vi "Insert Node.vi"(5 "Path to LabVIEW File":path, 6 "Variant in":variant, 7 "Shift Pressed?":bool, 8 "error in (no error)":errorcluster, 10 "QD Combo Box Ref":refnum<vi>, 11 "Selection List[]":refnum<vi>[](array[refnum])) -> (0 "error out":errorcluster, 3 "element":refnum<vi>, 4 "Variant out":variant)   [LabVIEW 2021, in "Migrator Reusables.lvlib"]
doc: "Inserts the object specified by name in the Quick Drop dialog box on the selected wire(s) on the diagram. If [Shift] is also pressed, and multiple wires were selected, a single instance of the object is inserted on those wires.\n\nDefault Shortcut - [I]"
uses:
  Migrator Reusables.lvlib
  <vilib>/Utility/miscctls.llb/LVPositionTypeDef.ctl
  <vilib>/Utility/miscctls.llb/LVPointTypeDef.ctl
  55ef8f48-70f1-403b-b4c9-42cfcc39d2a5.vi
  a401b57f-dff2-4459-b358-16b2136f329f.vi
  <vilib>/Comparison/Less/Less Functor/Less Functor.lvclass
panel:
  in  "Palette Object Name":string
  in  "Select a VI":string="Select a VI..."
  in  "Undo Name":string="Insert"
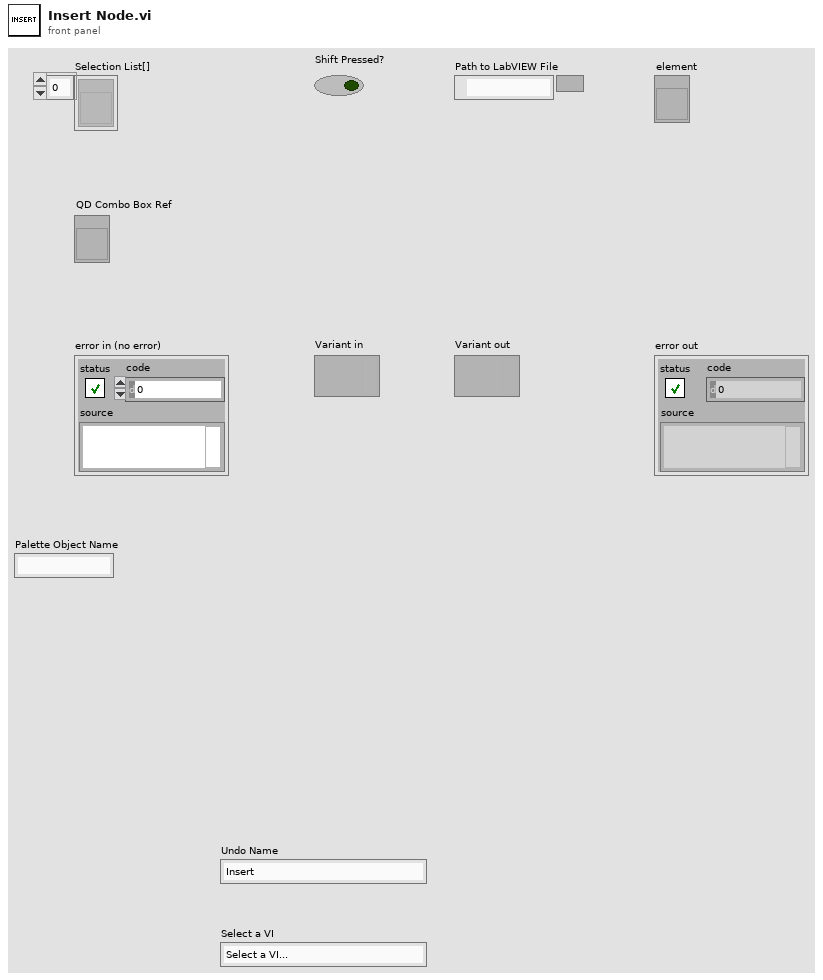
[diagram p1: front panel]
types:
  T1 = cluster{"Not Error Wire?":bool, "Source Term Top":i32, "Source Term Left":i32, "Wire Ref":refnum<vi>, "Source Term":refnum<vi>, "Sink Terms":refnum<vi>[], "Tried this one yet?":bool, "Sink Term Owner Owners":refnum<vi>[]}
  T2 = typedef "LVPositionTypeDef.ctl" = cluster{"Left":i32, "Top":i32}
  T3 = typedef "LVPointTypeDef.ctl" = cluster{"Horizontal":i16, "Vertical":i16}
  T4 = cluster{"Not Error Wire?":bool, "Source Term Top":i32, "Source Term Left":i32, "Wire Ref":refnum<vi>, "Source Term":refnum<vi>, "Sink Terms":refnum<vi>[], "Tried this one yet?":bool, "Sink Term Owner Owners":refnum<vi>[]}[]
  T5 = cluster{"Position":cluster{"h":i16, "v":i16}, "Flags":i32, "Type":enum32{"LooseEnd", "Endpoint", "Bend", "Junction"}, "Up Joint Index":i16, "Down Joint Index":i16, "Left Joint Index":i16, "Right Joint Index":i16}[]
  T6 = cluster{"Position":cluster{"h":i16, "v":i16}, "Flags":i32, "Type":enum32{"LooseEnd", "Endpoint", "Bend", "Junction"}, "Up Joint Index":i16, "Down Joint Index":i16, "Left Joint Index":i16, "Right Joint Index":i16}
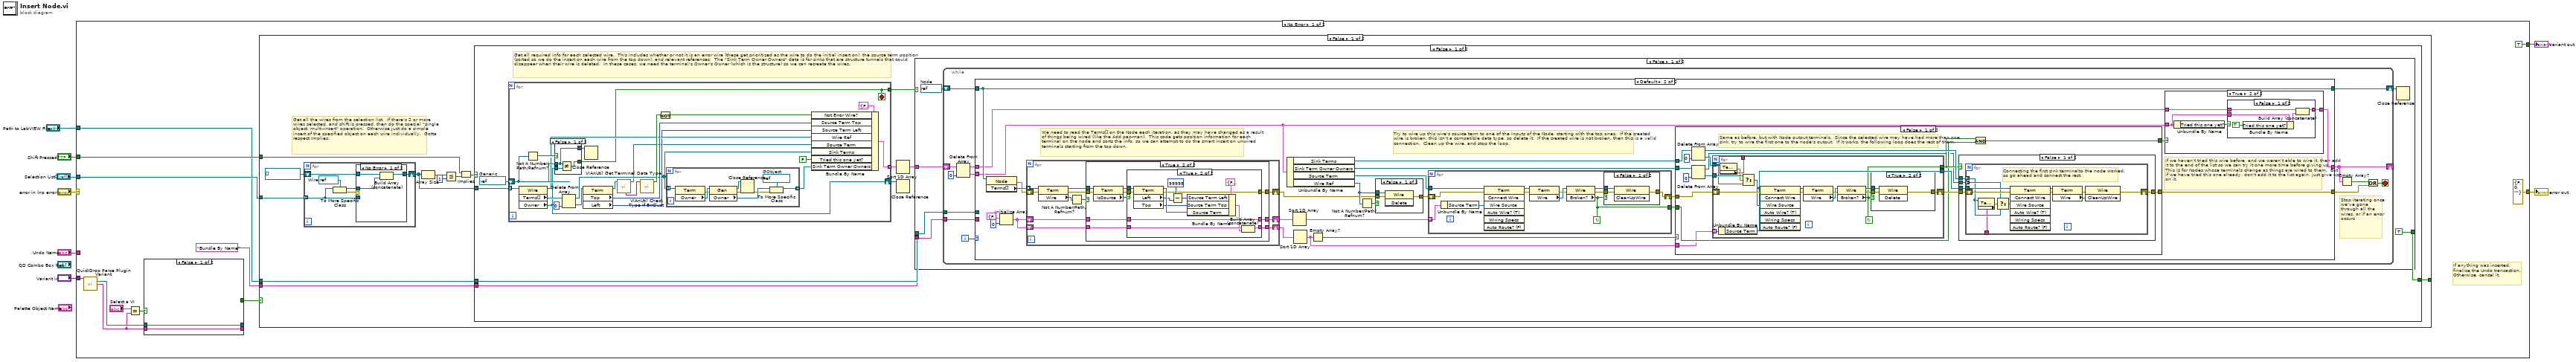
[diagram p0: block diagram]
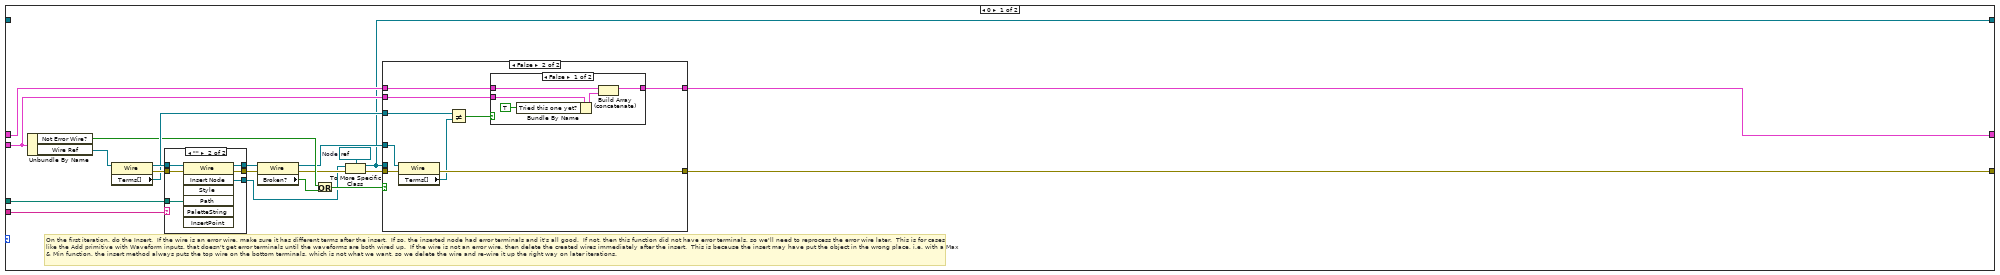
[diagram p2: hidden frame]
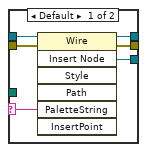
[diagram p3: hidden frame]
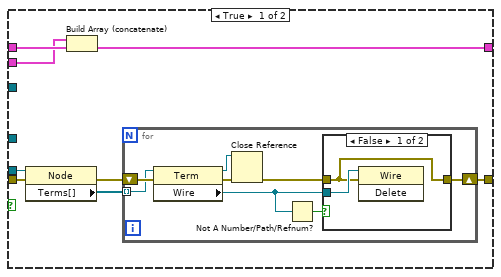
[diagram p4: hidden frame]
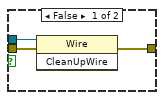
[diagram p9: hidden frame]
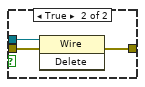
[diagram p13: hidden frame]
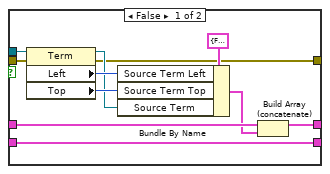
[diagram p15: hidden frame]
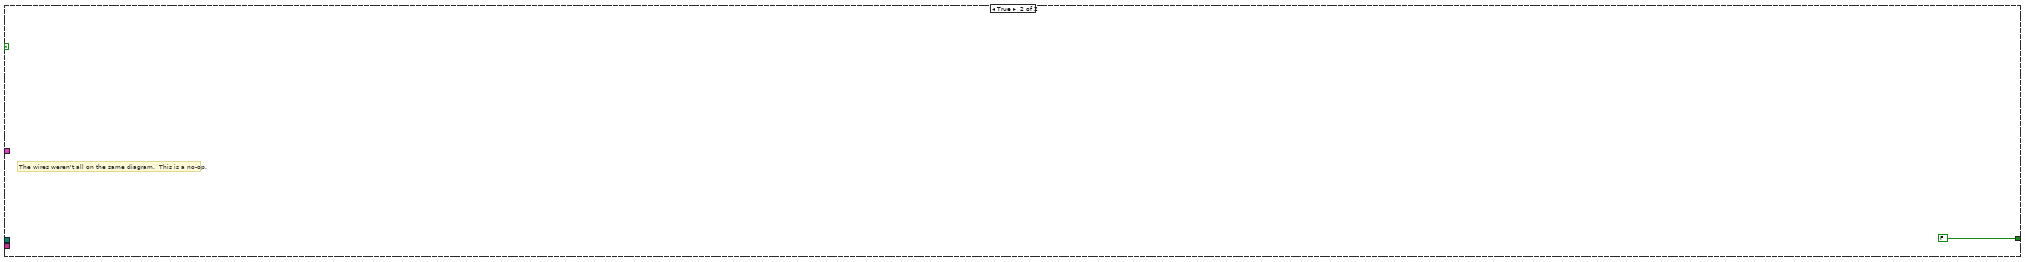
[diagram p16: hidden frame]
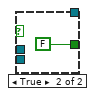
[diagram p17: hidden frame]
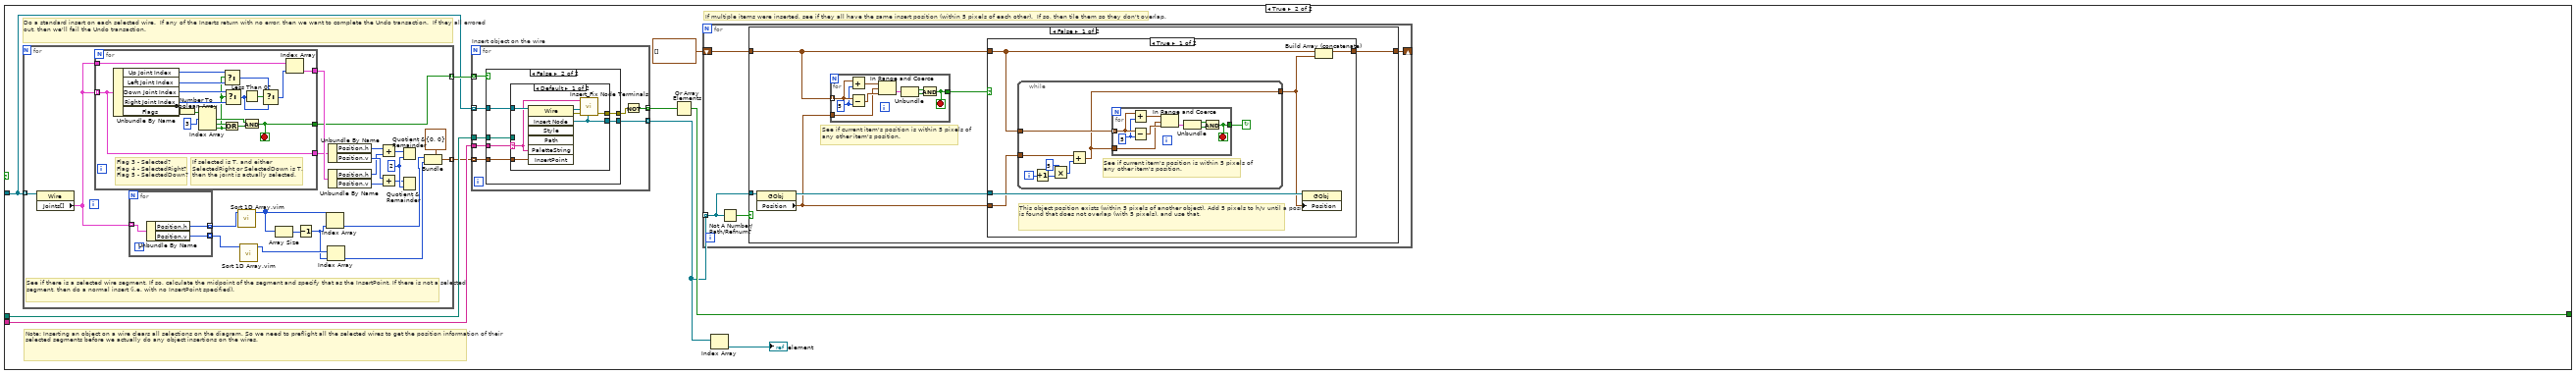
[diagram p18: hidden frame]
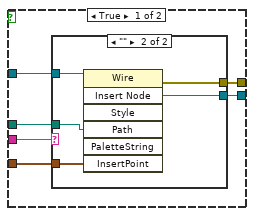
[diagram p19: hidden frame]
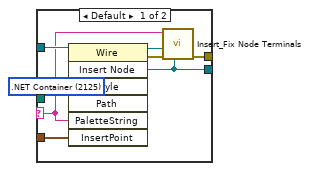
[diagram p20: hidden frame]
diagram:
  n1 = case shown="No Error" "error in (no error)" {
    selector: "error in (no error)" -> [_ w486]
    tunnel: [errorcluster {"status"=FALSE, "code"=0, "source"=""} ("error IO") w486] -> w7
    tunnel: "Shift Pressed?" -> [w18 _]
    tunnel: "Variant in" -> [w20 _]
    tunnel: "Undo Name" -> [_ _]
    tunnel: [TRUE _] -> w3
    tunnel: "Selection List[]" -> [w12 _]
    tunnel: "Path to LabVIEW File" -> [w9 _]
    frame No Error {
      # "If anything was inserted, finalize the Undo transaction.  Otherwise, cancel it."
      n2 = call <vilib>:"QuickDrop Parse Plugin Variant.vi"("QDKS Variant in"=w20) -> ("Project VI Path"=w15:path, "Palette Object Name"=w14:string)  [unwired: 12 in, 1 out]
      n3 = Equal?(x="Select a VI", y=w14) -> (x = y?=w16:bool)
      n4 = case shown="False" w16 {
        tunnel: w14 -> [w483 _]
        tunnel: w15 -> [w482 _]
        tunnel: [w483 _] -> _
        tunnel: [w482 w484] -> _
        tunnel: [_ w485] -> w13
        frame False {
        }
        frame True {
          # "NEW IN 2015: Catching \"Select a VI...\" and offering a file dialog to pick a VI to insert from disk."
          n5 = call <vilib>:"File Dialog - LabVIEW Files.vi"() -> ("cancelled"=w485:bool, "Path to LabVIEW File"=w484:path)  [unwired: 10 in]
        }
      }
      n6 = case shown="False" w13 {
        tunnel: w12 -> [w31 _]
        tunnel: w18 -> [w26 _]
        tunnel: [w23 _] -> _
        tunnel: w9 -> [w22 _]
        tunnel: "Bundle By Name" ("Palette Object Name") -> [w21 _]
        frame False {
          # "Get all the wires from the selection list.  If there's 2 or more wires selected, and shift is pressed, then do the special \"single object, multi-insert\" operation.  Otherwise just do a simple insert of the specified object on each wire individually.  Gotta respect Implies."
          n7 = for {
            tunnel: w31 -> [w473] mode=indexing
            shift-right: [w472] -> w25
            shift-left: refnum<vi>[] [] -> [w474]
            w476 = refnum<vi> refnum  # Wire
            n8 = To More Specific Class(target class=w476, reference=w473) -> (specific class reference=w471:refnum<vi>, error out=w475:errorcluster)  [unwired: 1 in]
            n9 = case shown="No Error" w475 {
              tunnel: w474 -> [w479 w481]
              tunnel: w473 -> [_ w480]
              tunnel: [w478 w481] -> w472
              tunnel: w471 -> [w477 _]
              frame No Error {
                n10 = Build Array (concatenate)(w479, w477) -> (w478:refnum<vi>[])
              }
              frame Error {
                n11 = Close Reference(reference=w480) -> ()  [unwired: 1 in, 1 out]
              }
            }
          }
          n12 = Array Size(array=w25) -> (size(s)=w29:i32)
          n13 = Less Or Equal?(x=w29, y=1) -> (x <= y?=w27:bool)
          n14 = Implies(1:w27, 2:w26) -> (0:w24:bool)
          n15 = case shown="False" w24 {
            tunnel: w21 -> [w33 w334]
            tunnel: w22 -> [w34 w333]
            tunnel: w25 -> [w36 w332]
            tunnel: [w32 w330] -> w23
            frame False {
              w39 = refnum<vi> refnum  # Generic
              # "Get all required info for each selected wire.  This includes whether or not it is an error wire (these get prioritized as the wire to do the initial insert on), the source term position (sorted so we do the insert on each wire from the top down), and relevant references.  The \"Sink Term Owner Owners\" data is for sinks that are structure tunnels that could disappear when their wire is deleted.  In these cases, we need the terminal's Owner's Owner (which is the structure) so we can recreate the wires."
              n16 = for {
                shift-right: [w298] -> w40
                shift-left: w39 -> [w313]
                tunnel: [w299] -> w38
                tunnel: w36 -> [w302] mode=indexing
                tunnel: [w301] -> w35 mode=indexing
                stop <- w299 stop-if-true
                n17 = property class="Wire"(reference=w302) -> (reference out=w305:refnum<vi>, "Terms[]"=w312:refnum<vi>[], "Owner"=w298:refnum<vi>)  [unwired: 1 in, 1 out]
                n18 = Not A Number/Path/Refnum?(number/path/refnum=w313) -> (NaN/Path/Refnum?=w310:bool)
                n19 = case shown="False" w310 {
                  tunnel: [w324 FALSE] -> w299
                  tunnel: w298 -> [w325 _]
                  tunnel: w313 -> [w323 _]
                  tunnel: [w323 _] -> w295
                  frame False {
                    n20 = Not Equal?(x=w323, y=w325) -> (x != y?=w324:bool)
                  }
                  frame True {
                  }
                }
                n21 = Delete From Array(array=w312, index=0) -> (deleted portion=w300:refnum<vi>, array with subset deleted=w297:refnum<vi>[])  [unwired: 1 in]
                n22 = property class="Term"(reference=w300) -> (reference out=w294:refnum<vi>, "Top"=w307:i32, "Left"=w296:i32)  [unwired: 1 in, 1 out]
                n23 = Close Reference(reference=w295) -> ()  [unwired: 1 in, 1 out]
                n24 = call <vilib>:"VIAnUtil Get Terminal Data Type.vi"("Terminal in"=w294) -> ("Terminal out"=w293:refnum<vi>, "Type Variant"=w292:variant)  [unwired: 7 in, 2 out]
                n25 = call <vilib>:"VIAnUtil Check Type If ErrClust.vi"("Data In"=w292) -> ("IsErrClust?"=w308:bool)  [unwired: 1 in, 9 out]
                n26 = Not(x=w308) -> (.not. x?=w306:bool)
                n27 = for {
                  tunnel: w297 -> [w322] mode=indexing
                  tunnel: [w319] -> w303 mode=indexing
                  w318 = refnum<vi> refnum  # GObject
                  n28 = property class="Term"(reference=w322) -> (error out=w317:errorcluster, "Owner"=w321:refnum<vi>)  [unwired: 1 in, 1 out]
                  n29 = property class="Gen"(reference=w321, error in=w317) -> (reference out=w315:refnum<vi>, error out=w316:errorcluster, "Owner"=w320:refnum<vi>)
                  n30 = Close Reference(reference=w315, error in (no error)=w316) -> (error out=w314:errorcluster)
                  n31 = To More Specific Class(target class=w318, reference=w320, error in=w314) -> (specific class reference=w319:refnum<vi>)  [unwired: 1 out]
                }
                n32 = Bundle By Name(cluster=T1 {"Not Error Wire?"=FALSE, "Source Term Top"=0, "Source Term Left"=0, "Wire Ref"=refnum, "Source Term"=refnum, "Sink Terms"=[], "Tried this one yet?"=FALSE, "Sink Term Owner Owners"=[]} ("Wire Information"), "Not Error Wire?"=w306, "Source Term Top"=w307, "Source Term Left"=w296, "Wire Ref"=w305, "Source Term"=w293, "Sink Terms"=w297, "Tried this one yet?"=FALSE, "Sink Term Owner Owners"=w303) -> (w301:T1)
              }
              n33 = Sort 1D Array(array=w35) -> (sorted array=w37:T4)
              n34 = Close Reference(reference=w40) -> ()  [unwired: 1 in, 1 out]
              n35 = case shown="False" w38 {
                tunnel: w37 -> [w46 _]
                tunnel: w33 -> [w43 _]
                tunnel: w34 -> [w42 _]
                tunnel: [TRUE FALSE] -> w32
                frame False {
                  w45 = refnum<vi> refnum  # Node
                  n36 = while {
                    shift-right: [w57] -> _
                    shift-left: w46 -> [w54]
                    shift-right: [w48] -> w44
                    shift-left: w45 -> [w56]
                    tunnel: w43 -> [w50]
                    tunnel: w42 -> [w49]
                    i -> [w58]
                    stop <- w51 stop-if-true
                    # "Stop iterating once we've gone through all the wires, or if an error occurs"
                    n37 = Delete From Array(array=w54, index=0) -> (deleted portion=w59:T1, array with subset deleted=w53:T4)  [unwired: 1 in]
                    n38 = case shown="Default" w58 {
                      tunnel: w59 -> [w79 w136]
                      tunnel: w53 -> [w67 w143]
                      tunnel: [w60 w151] -> w48
                      tunnel: [w80 w142] -> w57
                      tunnel: w56 -> [_ w151]
                      tunnel: [w78 w146] -> w47
                      tunnel: w50 -> [w65 _]
                      tunnel: w49 -> [w66 _]
                      frame 0 {
                        w63 = refnum<vi> refnum  # Node
                        # "On the first iteration, do the Insert.  If the wire is an error wire, make sure it has different terms after the insert.  If so, the inserted node had error terminals and it's all good.  If not, then this function did not have error terminals, so we'll need to reprocess the error wire later.  This is for cases like the Add primitive with Waveform inputs, that doesn't get error terminals until the waveforms are both wired up.  If the wire is not an error wire, then delete the created wires immediately after the insert.  This is because the insert may have put the object in the wrong place, i.e. with a Max & Min function, the insert method always puts the top wire on the bottom terminals, which is not what we want, so we delete the wire and re-wire it up the right way on later iterations."
                        n39 = Unbundle By Name(w79) -> ("Not Error Wire?"=w73:bool, "Wire Ref"=w77:refnum<vi>)
                        n40 = property class="Wire"(reference=w77) -> (reference out=w75:refnum<vi>, error out=w76:errorcluster, "Terms[]"=w74:refnum<vi>[])  [unwired: 1 in]
                        n41 = case shown="\"\"" w65 {
                          selector: w65 -> [w81 _]
                          tunnel: [w86 w92] -> w61
                          tunnel: w76 -> [w85 w91]
                          tunnel: w75 -> [w84 w90]
                          tunnel: [w83 w89] -> w72
                          tunnel: [w82 w88] -> w71
                          tunnel: w66 -> [_ w87]
                          frame Default {
                            n42 = invoke class="Wire" method="Insert Node"(reference=w84, error in=w85, "PaletteString"=w81) -> (reference out=w83:refnum<vi>, error out=w82:errorcluster, "Insert Node"=w86:refnum<vi>)  [unwired: 4 in, 4 out]
                          }
                          frame "" {
                            n43 = invoke class="Wire" method="Insert Node"(reference=w90, error in=w91, "Path"=w87) -> (reference out=w89:refnum<vi>, error out=w88:errorcluster, "Insert Node"=w92:refnum<vi>)  [unwired: 4 in, 4 out]
                          }
                        }
                        n44 = property class="Wire"(reference=w72, error in=w71) -> (reference out=w70:refnum<vi>, error out=w64:errorcluster, "Broken?"=w69:bool)
                        n45 = Or(x=w73, y=w69) -> (x .or. y?=w68:bool)
                        n46 = To More Specific Class(target class=w63, reference=w61, error in=w64) -> (specific class reference=w60:refnum<vi>, error out=w62:errorcluster)
                        n47 = case shown="False" w68 {
                          tunnel: w67 -> [w100 w120]
                          tunnel: [w98 w119] -> w80
                          tunnel: w79 -> [w99 w118]
                          tunnel: [w93 w115] -> w78
                          tunnel: w62 -> [w95 w117]
                          tunnel: w70 -> [_ w116]
                          tunnel: w74 -> [_ w113]
                          tunnel: w60 -> [w96 _]
                          frame True {
                            n48 = property class="Node"(reference=w96, error in=w95) -> (error out=w97:errorcluster, "Terms[]"=w94:refnum<vi>[])  [unwired: 1 out]
                            n49 = Build Array (concatenate)(w99, w100) -> (w98:T4)
                            n50 = for {
                              shift-right: [w102] -> w93
                              shift-left: w97 -> [w108]
                              tunnel: w94 -> [w107] mode=indexing
                              n51 = property class="Term"(reference=w107, error in=w108) -> (reference out=w105:refnum<vi>, error out=w106:errorcluster, "Wire"=w101:refnum<vi>)
                              n52 = Close Reference(reference=w105, error in (no error)=w106) -> (error out=w103:errorcluster)
                              n53 = Not A Number/Path/Refnum?(number/path/refnum=w101) -> (NaN/Path/Refnum?=w104:bool)
                              n54 = case shown="False" w104 {
                                tunnel: w103 -> [w109 w111]
                                tunnel: [w109 w111] -> w102
                                tunnel: w101 -> [w110 _]
                                frame False {
                                n55 = invoke class="Wire" method="Delete"(reference=w110, error in=w109) -> ()  [unwired: 1 in, 3 out]
                                }
                                frame True {
                                }
                              }
                            }
                          }
                          frame False {
                            n56 = property class="Wire"(reference=w116, error in=w117) -> (error out=w115:errorcluster, "Terms[]"=w114:refnum<vi>[])  [unwired: 1 out]
                            n57 = Not Equal?(x=w113, y=w114) -> (x != y?=w112:bool)
                            n58 = case shown="False" w112 {
                              tunnel: w120 -> [w125 w126]
                              tunnel: [w124 w126] -> w119
                              tunnel: w118 -> [w123 _]
                              frame False {
                                n59 = Bundle By Name(cluster=w123, "Tried this one yet?"=TRUE) -> (w122:T1)
                                n60 = Build Array (concatenate)(w125, w122) -> (w124:T4)
                              }
                              frame True {
                              }
                            }
                          }
                        }
                      }
                      frame Default {
                        # "If we haven't tried this wire before, and we weren't able to wire it, then add it to the end of the list so we can try it one more time before giving up.  This is for Nodes whose terminals change as things are wired to them.  But if we have tried this one already, don't add it to the list again, just give up on it."
                        # "Try to wire up this wire's source term to one of the inputs of the Node, starting with the top ones.  If the created wire is broken, this isn't a compatible data type, so delete it.  If the created wire is not broken, then this is a valid connection.  Clean up the wire, and stop the loop."
                        # "We need to read the Terms[] on the Node each iteration, as they may have changed as a result of things being wired (like the Add pac-man).  This code gets position information for each terminal on the node and sorts the info, so we can attempt to do the smart insert on unwired terminals starting from the top down."
                        n61 = property class="Node"(reference=w151) -> (error out=w129:errorcluster, "Terms[]"=w150:refnum<vi>[])  [unwired: 1 in, 1 out]
                        n62 = Initialize Array(T1 {"Not Error Wire?"=FALSE, "Source Term Top"=0, "Source Term Left"=0, "Wire Ref"=refnum, "Source Term"=refnum, "Sink Terms"=[], "Tried this one yet?"=FALSE, "Sink Term Owner Owners"=[]} ("Wire Information"), 0) -> (w130:T4)
                        n63 = for {
                          tunnel: w150 -> [w253] mode=indexing
                          shift-right: [w249] -> w148
                          shift-left: w130 -> [w252]
                          shift-right: [w248] -> w147
                          shift-left: w130 -> [w250]
                          shift-right: [w243] -> w128
                          shift-left: w129 -> [w245]
                          n64 = property class="Term"(reference=w253, error in=w245) -> (reference out=w246:refnum<vi>, error out=w244:errorcluster, "Wire"=w247:refnum<vi>)
                          n65 = Not A Number/Path/Refnum?(number/path/refnum=w247) -> (NaN/Path/Refnum?=w251:bool)
                          n66 = case shown="True" w251 {
                            tunnel: w252 -> [w256 w264]
                            tunnel: w250 -> [w255 w263]
                            tunnel: [w256 w261] -> w249
                            tunnel: [w255 w262] -> w248
                            tunnel: w246 -> [_ w266]
                            tunnel: w244 -> [w254 w259]
                            tunnel: [w254 w257] -> w243
                            frame False {
                            }
                            frame True {
                              n67 = property class="Term"(reference=w266, error in=w259) -> (reference out=w260:refnum<vi>, error out=w258:errorcluster, "IsSource"=w265:bool)
                              n68 = case shown="True" w265 {
                                tunnel: w264 -> [w276 w288]
                                tunnel: w263 -> [w277 w290]
                                tunnel: [w277 w289] -> w262
                                tunnel: [w275 w288] -> w261
                                tunnel: w260 -> [w272 w287]
                                tunnel: w258 -> [w268 w280]
                                tunnel: [w267 w279] -> w257
                                frame False {
                                n69 = property class="Term"(reference=w272, error in=w268) -> (reference out=w269:refnum<vi>, error out=w267:errorcluster, "Left"=w271:i32, "Top"=w270:i32)
                                n70 = Bundle By Name(cluster=T1 {"Not Error Wire?"=FALSE, "Source Term Top"=0, "Source Term Left"=0, "Wire Ref"=refnum, "Source Term"=refnum, "Sink Terms"=[], "Tried this one yet?"=FALSE, "Sink Term Owner Owners"=[]} ("Wire Information"), "Source Term Left"=w271, "Source Term Top"=w270, "Source Term"=w269) -> (w273:T1)
                                n71 = Build Array (concatenate)(w276, w273) -> (w275:T4)
                                }
                                frame True {
                                n72 = property class="Term"(reference=w287, error in=w280) -> (reference out=w284:refnum<vi>, error out=w279:errorcluster, "Left"=w278:i32, "Top"=w283:i32)
                                n73 = Subtract(x=99999, y=w278) -> (x-y=w281:i32)
                                n74 = Bundle By Name(cluster=T1 {"Not Error Wire?"=FALSE, "Source Term Top"=0, "Source Term Left"=0, "Wire Ref"=refnum, "Source Term"=refnum, "Sink Terms"=[], "Tried this one yet?"=FALSE, "Sink Term Owner Owners"=[]} ("Wire Information"), "Source Term Left"=w281, "Source Term Top"=w283, "Source Term"=w284) -> (w285:T1)
                                n75 = Build Array (concatenate)(w290, w285) -> (w289:T4)
                                }
                              }
                            }
                          }
                        }
                        n76 = Unbundle By Name(w136) -> ("Sink Terms"=w135:refnum<vi>[], "Sink Term Owner Owners"=w134:refnum<vi>[], "Source Term"=w132:refnum<vi>, "Wire Ref"=w131:refnum<vi>)
                        n77 = Sort 1D Array(array=w148) -> (sorted array=w141:T4)
                        n78 = Sort 1D Array(array=w147) -> (sorted array=w140:T4)
                        n79 = Empty Array?(array=w140) -> (empty?=w133:bool)
                        n80 = Not A Number/Path/Refnum?(number/path/refnum=w131) -> (NaN/Path/Refnum?=w139:bool)
                        n81 = case shown="False" w139 {
                          tunnel: [w153 w155] -> w149
                          tunnel: w131 -> [w154 _]
                          tunnel: w128 -> [w152 w155]
                          frame False {
                            n82 = invoke class="Wire" method="Delete"(reference=w154, error in=w152) -> (error out=w153:errorcluster)  [unwired: 1 in, 2 out]
                          }
                          frame True {
                          }
                        }
                        n83 = for {
                          tunnel: w132 -> [w236]
                          tunnel: w141 -> [w235] mode=indexing
                          tunnel: [w231] -> w144
                          shift-right: [w225] -> w127
                          shift-left: w149 -> [w229]
                          stop <- w231 continue-if-true
                          n84 = Unbundle By Name(w235) -> ("Source Term"=w230:refnum<vi>)
                          n85 = invoke class="Term" method="Connect Wire"(reference=w236, error in=w229, "Wire Source"=w230) -> (reference out=w234:refnum<vi>, error out=w228:errorcluster)  [unwired: 4 in, 5 out]
                          n86 = property class="Term"(reference=w234, error in=w228) -> (error out=w227:errorcluster, "Wire"=w233:refnum<vi>)  [unwired: 1 out]
                          n87 = property class="Wire"(reference=w233, error in=w227) -> (reference out=w232:refnum<vi>, error out=w226:errorcluster, "Broken?"=w231:bool)
                          n88 = case shown="False" w231 {
                            tunnel: w232 -> [w239 w242]
                            tunnel: w226 -> [w238 w241]
                            tunnel: [w237 w240] -> w225
                            frame False {
                              n89 = invoke class="Wire" method="CleanUpWire"(reference=w239, error in=w238) -> (error out=w237:errorcluster)  [unwired: 1 in, 2 out]
                            }
                            frame True {
                              n90 = invoke class="Wire" method="Delete"(reference=w242, error in=w241) -> (error out=w240:errorcluster)  [unwired: 1 in, 2 out]
                            }
                          }
                        }
                        n91 = case shown="False" w133 {
                          tunnel: w135 -> [w171 _]
                          tunnel: [w165 w212] -> w146
                          tunnel: [w164 w213] -> w145
                          tunnel: w144 -> [w162 w213]
                          tunnel: w134 -> [w160 _]
                          tunnel: w140 -> [w157 _]
                          tunnel: w127 -> [w156 w212]
                          frame False {
                            # "Same as before, but with Node output terminals.  Since the selected wire may have had more than one sink, try to wire the first one to the node's output.  If it works, the following loop does the rest of them."
                            n92 = Delete From Array(array=w171, index=0) -> (deleted portion=w169:refnum<vi>, array with subset deleted=w166:refnum<vi>[])  [unwired: 1 in]
                            n93 = Delete From Array(array=w160, index=0) -> (deleted portion=w159:refnum<vi>, array with subset deleted=w158:refnum<vi>[])  [unwired: 1 in]
                            n94 = for {
                              tunnel: w169 -> [w191]
                              tunnel: w157 -> [w196] mode=indexing
                              shift-right: [w198] -> w168
                              shift-left: w156 -> [w205]
                              tunnel: [w193] -> w163
                              tunnel: [w194] -> w167
                              tunnel: w159 -> [w197]
                              tunnel: [w190] -> _
                              stop <- w193 continue-if-true
                              n95 = Unbundle By Name(w196) -> ("Source Term"=w194:refnum<vi>)
                              n96 = property class="Term"(reference=w191) -> (error out=w192:errorcluster, "ClassName"=w190:string)  [unwired: 1 in, 1 out]
                              n97 = Select(t=w197, s=w192, f=w191) -> (s? t:f=w195:refnum<vi>)
                              n98 = invoke class="Term" method="Connect Wire"(reference=w194, error in=w205, "Wire Source"=w195) -> (reference out=w203:refnum<vi>, error out=w204:errorcluster)  [unwired: 4 in, 5 out]
                              n99 = property class="Term"(reference=w203, error in=w204) -> (error out=w202:errorcluster, "Wire"=w201:refnum<vi>)  [unwired: 1 out]
                              n100 = property class="Wire"(reference=w201, error in=w202) -> (reference out=w199:refnum<vi>, error out=w200:errorcluster, "Broken?"=w193:bool)
                              n101 = case shown="True" w193 {
                                tunnel: w200 -> [w208 w210]
                                tunnel: w199 -> [w207 w211]
                                tunnel: [w206 w209] -> w198
                                frame False {
                                n102 = invoke class="Wire" method="CleanUpWire"(reference=w207, error in=w208) -> (error out=w206:errorcluster)  [unwired: 1 in, 2 out]
                                }
                                frame True {
                                n103 = invoke class="Wire" method="Delete"(reference=w211, error in=w210) -> (error out=w209:errorcluster)  [unwired: 1 in, 2 out]
                                }
                              }
                            }
                            n104 = case shown="False" w163 {
                              tunnel: w168 -> [w176 w189]
                              tunnel: [w173 w189] -> w165
                              tunnel: w167 -> [w175 _]
                              tunnel: w166 -> [w174 _]
                              tunnel: w158 -> [w172 _]
                              frame False {
                                n105 = for {
                                tunnel: w175 -> [w187]
                                tunnel: w174 -> [w179] mode=indexing
                                shift-right: [w177] -> w173
                                shift-left: w176 -> [w188]
                                tunnel: w172 -> [w182] mode=indexing
                                tunnel: [w178] -> _
                                # "Connecting the first sink terminalto the node worked, so go ahead and connect the rest."
                                n106 = property class="Term"(reference=w179) -> (error out=w180:errorcluster, "ClassName"=w178:string)  [unwired: 1 in, 1 out]
                                n107 = Select(t=w182, s=w180, f=w179) -> (s? t:f=w181:refnum<vi>)
                                n108 = invoke class="Term" method="Connect Wire"(reference=w187, error in=w188, "Wire Source"=w181) -> (reference out=w186:refnum<vi>, error out=w185:errorcluster)  [unwired: 4 in, 5 out]
                                n109 = property class="Term"(reference=w186, error in=w185) -> (error out=w184:errorcluster, "Wire"=w183:refnum<vi>)  [unwired: 1 out]
                                n110 = invoke class="Wire" method="CleanUpWire"(reference=w183, error in=w184) -> (error out=w177:errorcluster)  [unwired: 1 in, 2 out]
                                }
                              }
                              frame True {
                                # "None of the node outputs would connect to this wire.  No need to try to process the rest of the sinks."
                              }
                            }
                            n111 = And(x=w163, y=w162) -> (x .and. y?=w164:bool)
                          }
                          frame True {
                            # "There are no more unwired outputs on the node.  Don't bother trying to find one to wire to."
                          }
                        }
                        n112 = case shown="True" w145 {
                          tunnel: w143 -> [w214 w218]
                          tunnel: w136 -> [_ w215]
                          tunnel: [w214 w216] -> w142
                          frame False {
                          }
                          frame True {
                            n113 = Unbundle By Name(w215) -> ("Tried this one yet?"=w217:bool)
                            n114 = case shown="False" w217 {
                              tunnel: w218 -> [w223 w224]
                              tunnel: [w222 w224] -> w216
                              tunnel: w215 -> [w221 _]
                              frame False {
                                n115 = Bundle By Name(cluster=w221, "Tried this one yet?"=TRUE) -> (w220:T1)
                                n116 = Build Array (concatenate)(w223, w220) -> (w222:T4)
                              }
                              frame True {
                              }
                            }
                          }
                        }
                      }
                    }
                    n117 = Empty Array?(array=w57) -> (empty?=w52:bool)
                    n118 = Or(x=w52, y=w47) -> (x .or. y?=w51:bool)
                  }
                  n119 = Close Reference(reference=w44) -> ()  [unwired: 1 in, 1 out]
                }
                frame True {
                  # "The wires weren't all on the same diagram.  This is a no-op."
                }
              }
            }
            frame True {
              # "Note: Inserting an object on a wire clears all selections on the diagram. So we need to preflight all the selected wires to get the position information of their selected segments before we actually do any object insertions on the wires."
              # "If multiple items were inserted, see if they all have the same insert position (within 5 pixels of each other).  If so, then tile them so they don't overlap."
              # "Do a standard insert on each selected wire.  If any of the Inserts return with no error, then we want to complete the Undo transaction.  If they all errored out, then we'll fail the Undo transaction."
              n120 = for {
                tunnel: w332 -> [w448] mode=indexing
                tunnel: [w437] -> w335 mode=indexing
                tunnel: [w436] -> w327 mode=indexing
                w443 = i16 2 ("y")
                # "See if there is a selected wire segment. If so, calculate the midpoint of the segment and specify that as the InsertPoint. If there is not a selected segment, then do a normal insert (i.e. with no InsertPoint specified)."
                n121 = property class="Wire"(reference=w448) -> ("Joints[]"=w435:T5)  [unwired: 1 in, 2 out]
                n122 = for {
                  tunnel: w435 -> [w464] mode=indexing
                  tunnel: w435 -> [w463]
                  tunnel: [w464] -> w439
                  tunnel: [w462] -> w440
                  tunnel: [w452] -> w437
                  stop <- w452 stop-if-true
                  # "If selected is T, and either SelectedRight or SelectedDown is T, then the joint is actually selected."
                  # "Flag 3 - Selected?\nFlag 4 - SelectedRight?\nFlag 5 - SelectedDown?"
                  n123 = Unbundle By Name(w464) -> ("Up Joint Index"=w459:i16, "Left Joint Index"=w458:i16, "Down Joint Index"=w461:i16, "Right Joint Index"=w460:i16, "Flags"=w470:i32)
                  n124 = Number To Boolean Array(number=w470) -> (Boolean array=w469:bool[])
                  n125 = Index Array(array=w469, index #1=3 ("index")) -> (element #1=w465:bool, element #2=w466:bool, element #3=w457:bool)  [unwired: 2 in]
                  n126 = Select(t=w459, s=w457, f=w458) -> (s? t:f=w454:i16)
                  n127 = Or(x=w466, y=w457) -> (x .or. y?=w467:bool)
                  n128 = Select(t=w461, s=w457, f=w460) -> (s? t:f=w453:i16)
                  n129 = Less Than 0?(x=w453) -> (x < 0?=w455:bool)
                  n130 = And(x=w465, y=w467) -> (x .and. y?=w452:bool)
                  n131 = Select(t=w454, s=w455, f=w453) -> (s? t:f=w456:i16)
                  n132 = Index Array(array=w463, index=w456) -> (element=w462:T6)
                }
                n133 = for {
                  tunnel: w435 -> [w451] mode=indexing
                  tunnel: [w450] -> w433 mode=indexing
                  tunnel: [w449] -> w432 mode=indexing
                  n134 = Unbundle By Name(w451) -> ("Position.h"=w450:i16, "Position.v"=w449:i16)
                }
                n135 = call "Sort 1D Array.vim"("unsorted array"=w433) -> ("sorted array"=w431:i16[])  [unwired: 10 in]
                n136 = call "Sort 1D Array.vim"("unsorted array"=w432) -> ("sorted array"=w429:i16[])  [unwired: 10 in]
                n137 = Array Size(array=w431) -> (size(s)=w430:i32)
                n138 = Decrement(x=w430) -> (x-1=w428:i32)
                n139 = Index Array(array=w431, index=w428) -> (element=w434:i16)
                n140 = Index Array(array=w429, index=w428) -> (element=w427:i16)
                n141 = Unbundle By Name(w439) -> ("Position.h"=w444:i16, "Position.v"=w446:i16)
                n142 = Unbundle By Name(w440) -> ("Position.h"=w445:i16, "Position.v"=w447:i16)
                n143 = Add(x=w444, y=w445) -> (x+y=w441:i16)
                n144 = Add(x=w446, y=w447) -> (x+y=w442:i16)
                n145 = Quotient & Remainder(x=w441, y=w443) -> ()  [unwired: 2 out]
                n146 = Quotient & Remainder(x=w442, y=w443) -> ()  [unwired: 2 out]
                n147 = Bundle(cluster=T3 {"Horizontal"=0, "Vertical"=0} ("Insertion Point"), "Horizontal"=w434, "Vertical"=w427) -> (w436:T3)
              }
              n148 = for "Insert object on the wire" {
                tunnel: w335 -> [w344] mode=indexing
                tunnel: w334 -> [w343]
                tunnel: w333 -> [w342]
                tunnel: w332 -> [w341] mode=indexing
                tunnel: [w340] -> w329 mode=indexing
                tunnel: [w338] -> w331 mode=indexing
                tunnel: w327 -> [w337] mode=indexing
                n149 = case shown="False" w344 {
                  tunnel: w343 -> [w350 w369]
                  tunnel: w342 -> [w349 w368]
                  tunnel: [w348 w367] -> w340
                  tunnel: w341 -> [w347 w366]
                  tunnel: [w346 w365] -> w339
                  tunnel: w337 -> [w345 w364]
                  frame True {
                    n150 = case shown="\"\"" w350 {
                      selector: w350 -> [w354 _]
                      tunnel: w347 -> [w358 w363]
                      tunnel: w349 -> [_ w362]
                      tunnel: [w357 w361] -> w346
                      tunnel: [w356 w360] -> w348
                      tunnel: w345 -> [w351 w359]
                      frame Default {
                        w352 = 2125 items=[".NET Container"=2125, ".NET Refnum"=3441, "2D Picture"=3508, "3D Picture"=23776, "Absolute Value"=1054, "Accept TLS"=1732, "Access Rights"=1412, "ActiveX Container"=2072, "Add"=1050, "Add (with error terminals)"=3915, "Add Array Elements"=1903, "Add Entropy"=1738, "Add Private Key To TLS Configuration"=1735, "Add Trusted Certificate To TLS Configuration"=1736, "Agitator"=3831, "AllSpoll"=1960, "Always Copy"=2400, "And"=1061, "And Array Elements"=1911, "Append True/False String"=1511, "Application Refnum"=3412, "Array (block diagram constant)"=2070, "Array (classic)"=3300, "Array (modern)"=21608, "Array Interface Control"=23777, "Array Max & Min"=1907, "Array of Strings to Path"=1422, "Array Size"=1809, "Array Subset"=2044, "Array To Cluster"=1168, "Array To Spreadsheet String"=1540, "ArrayMemInfo"=2412, "Assert Structural Type Match"=2416, "Assert Structural Type Mismatch"=2464, "Atmospheric Tank (classic)"=3070, "Atmospheric Tank (modern)"=21751, "Automation Close"=8001, "Automation Open"=8000, "Automation Refnum"=3410, "Avogadro Constant (1/mol)"=23520, "Base 10 Logarithm Of e"=23512, "Bin #1"=3073, "Bin #2"=21755, "Bitpack to Array"=3135, "Bluetooth Close Connection"=9148, "Bluetooth Create Listener"=9151, "Bluetooth Discover"=9152, "Bluetooth Network Connection Refnum"=3468, "Bluetooth Open Connection"=9153, "Bluetooth Read"=9149, "Bluetooth Wait On Listener"=9147, "Bluetooth Write"=9150, "Boolean Array To Number"=1815, "Boolean To (0,1)"=1167, "Build Array"=2041, "Build Cluster Array"=2047, "Build Map"=2463, "Build Matrix"=8500, "Build Path"=1419, "Build Set"=2462, "Build Waveform"=2066, "Bundle"=2049, "Bundle By Name"=2057, "Byte Array To String"=1609, "Byte Array To UTF-8 String"=1651, "Byte Stream File Refnum"=3408, "Call By Reference"=3901, "Call Chain"=1999, "Call Library Function Node"=2062, "Call MATLAB Function"=24210, "Call Parent Class Method"=2354, "CAN Channel (block diagram constant)"=2124, "CAN Channel (classic)"=3340, "CAN Channel (modern)"=21817, "CAN Channel (system)"=21966, "CAN Interface (block diagram constant)"=2123, "CAN Interface (classic)"=3339, "CAN Interface (modern)"=21815, "CAN Interface (system)"=21964, "CAN Task (block diagram constant)"=3471, "CAN Task (classic)"=3470, "CAN Task (modern)"=21789, "CAN Task (system)"=21963, "Cancel Button (modern)"=21739, "Cancel Button (system)"=3131, "Cancel Notification"=9107, "Carriage Return Constant"=23500, "Case Structure"=2001, "Cast Unit Bases"=1079, "Check Valve"=3833, "Checkbox (classic)"=3117, "CheckBox (modern)"=21924, "Checkbox (system)"=3132, "Class Specifier Constant"=2094, "Classic Color Box"=3013, "Classic Color Ramp"=3022, "Classic Horizontal Slide Switch"=3114, "Classic Vertical Slide"=3004, "Clear Fixed-Point Overflow Status"=5562, "Close File"=8052, "Close File (deprecated)"=1405, "Close MATLAB Session"=24209, "Close Python Session"=24207, "Close Reference"=8011, "Close TLS Configuration"=1741, "Close Variable Connection"=23783, "Closure Structure"=2372, "Cluster (classic)"=3400, "Cluster (modern)"=21607, "Cluster Constant"=2071, "Cluster To Array"=1169, "Code Interface Node"=2050, "Coerce To Type"=2402, "Collection Size"=2450, "Color Box Constant"=2120, "Color Box Thin Border"=2905, "Colored Rectangle (broken?)"=3625, "Combo Box (classic)"=3304, "Combo Box (modern)"=21604, "Combo Box (system)"=21917, "Combo Box Constant"=2088, "Complex Conjugate"=1048, "Complex To Polar"=1045, "Complex To Re/Im"=1044, "Compound Arithmetic"=2200, "Compressor"=3832, "Concatenate Strings"=2040, "Conditional Disable Structure"=2064, "Constructor Node"=3904, "Control & Simulation Loop"=2099, "Control Help Window"=1353, "Control Online Help"=1355, "Control Refnum"=3419, "Convert Unit"=2059, "Conveyer"=3827, "Copy"=8053, "Copy (deprecated)"=1416, "Cosecant"=1204, "Cosine"=1201, "Cotangent"=1205, "CPU Information"=24130, "Create Folder"=8055, "Create Network Stream Endpoint"=23793, "Create Network Stream Reader Endpoint"=23811, "Create Network Stream Writer Endpoint"=23810, "Create Stream"=23796, "Create Unique Network Stream Endpoint"=23795, "Create Unique Network Stream Reader Endpoint"=23807, "Create Unique Network Stream Writer Endpoint"=23806, "Create User Event"=2073, "Current Processor ID"=24131, "Current VI's Menubar"=9000, "Current VI's Path"=1426, "DAQmx Analog Trigger Source (block diagram constant)"=2119, "DAQmx Analog Trigger Source (classic)"=3336, "DAQmx Analog Trigger Source (modern)"=21774, "DAQmx Analog Trigger Source (system)"=21951, "DAQmx Device Name (block diagram constant)"=2093, "DAQmx Device Name (classic)"=3318, "DAQmx Device Name (modern)"=21773, "DAQmx Device Name (system)"=21950, "DAQmx Global Channel (block diagram constant)"=3430, "DAQmx Global Channel (classic)"=3443, "DAQmx Global Channel (modern)"=21770, "DAQmx Global Channel (system)"=21957, "DAQmx Physical Channel (block diagram constant)"=2118, "DAQmx Physical Channel (classic)"=3335, "DAQmx Physical Channel (modern)"=21777, "DAQmx Physical Channel (system)"=21954, "DAQmx Scale Name (block diagram constant)"=2116, "DAQmx Scale Name (classic)"=3317, "DAQmx Scale Name (modern)"=21775, "DAQmx Scale Name (system)"=21952, "DAQmx Switch (block diagram constant)"=2121, "DAQmx Switch (classic)"=3337, "DAQmx Switch (modern)"=21776, "DAQmx Switch (system)"=21953, "DAQmx Task Name (block diagram constant)"=3434, "DAQmx Task Name (classic)"=3442, "DAQmx Task Name (modern)"=21778, "DAQmx Task Name (system)"=21959, "DAQmx Terminal (block diagram constant)"=2117, "DAQmx Terminal (classic)"=3319, "DAQmx Terminal (modern)"=21781, "DAQmx Terminal (system)"=21955, "Data Cache Size"=24132, "Data Log File Refnum"=3402, "Data Value Reference"=3476, "Data Value Reference Constant"=24134, "DataSocket Close"=1085, "DataSocket Open"=1084, "DataSocket Read"=1086, "DataSocket Refnum"=3417, "DataSocket Write"=1087, "Date/Time To Seconds"=1308, "Decimal Digit?"=1119, "Decimal String To Number"=1184, "Decimate 1D Array"=2046, "DecomposeLockDataValRef"=2406, "DecomposeVariant"=2404, "Decrement"=1058, "Default Directory"=1427, "Delete"=8056, "Delete (deprecated)"=1417, "Delete Data Value Reference"=2409, "Delete From Array"=3912, "Delete Menu Items"=9004, "Delete Variant Attribute"=8206, "Delete Waveform Attribute"=8209, "Deny Access"=8057, "Dequeue Element"=9113, "Destroy Stream Endpoint"=23794, "Destroy User Event"=2075, "DevClear"=1961, "DevClearList"=1962, "Device Control/Status"=1433, "Device Refnum"=3405, "Diagram Disable Structure"=2054, "Dial (classic)"=3050, "Dial (modern)"=21732, "Digital Data (classic)"=3210, "Digital Data (modern)"=21216, "Digital Waveform Graph (classic)"=3511, "Digital Waveform Graph (modern)"=21718, "Direct Variable Read"=23785, "Direct Variable Write"=23788, "Divide"=1053, "Divide (with error terminals)"=3918, "Dlg Horiz Scrollbar"=21905, "Dlg Mac Group Box"=32514, "Dlg Numeric #1"=2100, "Dlg Numeric #2"=3006, "Dlg String"=2110, "Dlg Vert Scrollbar"=21906, "Down Arrow"=3824, "Down Bow Valve (flat)"=3707, "Down Bow Valve (outline)"=3807, "Down Bow Valve (shaded)"=21767, "Down Rect Valve (flat)"=3706, "Down Rect Valve (outline)"=3806, "Down Rect Valve (shaded)"=21766, "Down Tee (flat)"=3818, "Down Tee (shaded)"=3718, "Dynamic FPGA Interface Cast"=5690, "Eased Corner Rectangle"=32513, "Element of Set?"=2454, "Elementary Charge (C)"=23517, "Empty Array?"=23063, "Empty Collection?"=2451, "Empty Path Constant"=23523, "Empty String Constant"=23503, "Empty String/Path?"=1112, "Enable Menu Tracking"=9002, "EnableLocal"=1963, "EnableRemote"=1964, "End of Line Constant"=23525, "Enqueue Element"=9111, "Enqueue Element At Opposite End"=9129, "Enum (classic)"=3023, "Enum (modern)"=21605, "Enum (system)"=3062, "Enum Constant"=2090, "EOF"=1410, "Equal To 0?"=1113, "Equal?"=1102, "Error Ring Constant"=2039, "Event Callback Refnum"=3435, "Event Data Node"=2102, "Event Structure"=2052, "Exchanger"=3828, "Exclusive Or"=1063, "Exponential"=1211, "Exponential (Arg) -1"=1222, "Expression Node"=2201, "False Constant"=2006, "Feedback Node"=2353, "FieldPoint IO Point (block diagram constant)"=3440, "FieldPoint IO Point (classic)"=3439, "FieldPoint IO Point (modern)"=21784, "FIFO Refnum"=3474, "File Dialog"=8058, "File Dialog (deprecated)"=8081, "File Path Control (classic)"=3203, "File Path Control (modern)"=21730, "File Path Control (system)"=21922, "File Path Indicator (classic)"=3204, "File Path Indicator (modern)"=21731, "File/Directory Info"=8082, "File/Directory Info (deprecated)"=1413, "FindLstn"=1965, "FindRQS"=1966, "First Call?"=1083, "Fixed-Point Overflow?"=5565, "Fixed-Point to Integer Cast"=5566, "Flat Box"=3602, "Flat Circle"=3605, "Flat Down Triangle"=3623, "Flat Frame"=3608, "Flat Left Triangle"=3620, "Flat Right Triangle"=3621, "Flat Round Button"=3102, "Flat Rounded Box"=3611, "Flat Sequence Structure"=2069, "Flat Square Button"=3103, "Flat Up Triangle"=3622, "Flatten To JSON"=24201, "Flatten To String"=1164, "Flatten To XML"=8402, "Flattened String To Variant"=8202, "Floating Point Equal?"=23064, "Flush Event Queue"=2135, "Flush File"=8059, "Flush File (deprecated)"=1406, "Flush Queue"=9114, "Flush Stream"=23808, "For Loop"=2002, "Fork"=2194, "Format Date/Time String"=8100, "Format Into File"=2083, "Format Into String"=2081, "Format Value"=1512, "Formula Node"=2004, "FPGA Refnum to Session"=2322, "Fract/Exp String To Number"=1187, "Framed Color Box (classic)"=3008, "Framed Color Box (modern)"=21019, "Free Label"=2321, "Furnace"=3829, "Gauge (classic)"=3040, "Gauge (modern)"=21009, "Gauge for Simon"=32600, "Generate Front Panel Activity"=1329, "Generate Occurrence"=1700, "Generate User Event"=2074, "Generate User-Defined Trace Event"=2250, "Get Control Values by Index"=24204, "Get Datalog Position"=8061, "Get Date/Time In Seconds"=1303, "Get Date/Time String"=1600, "Get Drag Drop Data"=9154, "Get File Position"=8062, "Get File Size"=8063, "Get Fixed-Point Components"=11163, "Get Help Window Status"=1354, "Get Matrix Diagonal"=8501, "Get Matrix Elements"=8502, "Get Menu Item Info"=9005, "Get Menu Selection"=9001, "Get Menu Short Cut Info"=9007, "Get Notifier Status"=9103, "Get Number of Records"=8064, "Get Permissions"=8065, "Get Queue Status"=9110, "Get Submatrix"=8503, "Get Type and Creator"=8066, "Get Variant Attribute"=8205, "Get Volume Info"=8067, "Get Waveform Attribute"=8208, "Get Waveform Components"=2067, "Global Variable"=2060, "GPIB Clear"=1954, "GPIB Initialization"=1957, "GPIB Misc"=1956, "GPIB Read"=1951, "GPIB Serial Poll"=1955, "GPIB Status"=1959, "GPIB Trigger"=1953, "GPIB Wait"=1958, "GPIB Write"=1950, "Gravitational Constant (N m2/kg2)"=23519, "Greater Or Equal To 0?"=1114, "Greater Or Equal?"=1103, "Greater Than 0?"=1117, "Greater?"=1110, "Handle Peek"=1604, "Handle Poke"=1605, "Hex Digit?"=1123, "Hexadecimal String To Number"=1185, "Hopper #1"=21754, "Hopper #2"=3072, "Horiz Line"=3821, "Horiz Pipe (flat)"=3810, "Horiz Pipe (shaded)"=3710, "Horizontal Button Box"=3636, "Horizontal Fill Slide (classic)"=3012, "Horizontal Fill Slide (modern)"=21100, "Horizontal Gradient Oval"=32502, "Horizontal Gradient Rectangle"=32504, "Horizontal Gradient Rounded Rectangle"=32507, "Horizontal Graduated Bar"=21106, "Horizontal Pointer Slide (classic)"=3011, "Horizontal Pointer Slide (modern)"=21101, "Horizontal Pointer Slide (system)"=21902, "Horizontal Progress Bar (modern)"=21102, "Horizontal Progress Bar (system)"=21910, "Horizontal Scrollbar"=21110, "Horizontal Slide (classic)"=3010, "Horizontal Slide (system)"=21904, "Horizontal Smooth Box"=3633, "Horizontal Splitter Bar"=21861, "Horizontal Splitter Bar (Classic)"=21863, "Horizontal Splitter Bar (NXG Style)"=21867, "Horizontal Splitter Bar (System)"=21865, "Horizontal Switch"=3108, "Horizontal Tank"=3071, "Horizontal Toggle Switch (classic)"=3110, "Horizontal Toggle Switch (modern)"=21700, "Hyperbolic Cosecant"=23053, "Hyperbolic Cosine"=1215, "Hyperbolic Cotangent"=23055, "Hyperbolic Secant"=23054, "Hyperbolic Sine"=1214, "Hyperbolic Tangent"=1216, "IMAQ Session"=3415, "Implies"=1080, "In Place Element Structure"=2360, "In Range and Coerce"=1127, "Include Fixed-Point Overflow Status"=5564, "Increment"=1057, "Index & Bundle Cluster Array"=2056, "Index Array"=2042, "Index String Array"=1531, "Initialize Array"=2053, "Inline C Node"=2104, "Insert Into Array"=3911, "Insert Into Map"=2456, "Insert Into Set"=2452, "Insert Menu Items"=9003, "Integer to Fixed-Point Cast"=5567, "Intensity Chart (classic)"=3509, "Intensity Chart (modern)"=21719, "Intensity Graph (classic)"=3510, "Intensity Graph (modern)"=21720, "Interleave 1D Arrays"=2045, "Interpolate 1D Array"=1905, "Inverse Cosecant"=23050, "Inverse Cosine"=1207, "Inverse Cotangent"=23052, "Inverse Hyperbolic Cosecant"=23056, "Inverse Hyperbolic Cosine"=1218, "Inverse Hyperbolic Cotangent"=23058, "Inverse Hyperbolic Secant"=23057, "Inverse Hyperbolic Sine"=1217, "Inverse Hyperbolic Tangent"=1219, "Inverse Secant"=23051, "Inverse Sine"=1206, "Inverse Tangent"=1208, "Inverse Tangent (2 Input)"=1228, "Invoke Node"=3900, "IP To String"=1710, "IrDA Close Connection"=9144, "IrDA Create Listener"=9140, "IrDA Discover"=9141, "IrDA Network Connection Refnum"=3450, "IrDA Open Connection"=9142, "IrDA Read"=9145, "IrDA Wait On Listener"=9143, "IrDA Write"=9146, "IsDebuggingActive"=2403, "IVI Delete Session"=8103, "IVI Logical Name (block diagram constant)"=3420, "IVI Logical Name (classic)"=3414, "IVI Logical Name (modern)"=21736, "IVI New Session"=8102, "Join"=2195, "Join Numbers"=1171, "Junction"=2197, "Knob (classic)"=3005, "Knob (modern)"=21000, "Label (modern)"=21960, "Label (system)"=21961, "Labeled Oblong Button"=3125, "Labeled Rectangular Button"=3124, "Labeled Round Button"=3122, "Labeled Square Button"=3123, "LabVIEW Object"=3457, "Leak Variant Value Reference"=2410, "LED Button"=3116, "Left Arrow"=3826, "Left Bow Valve (flat)"=3701, "Left Bow Valve (outline)"=3801, "Left Bow Valve (shaded)"=21761, "Left Down Elbow (flat)"=3811, "Left Down Elbow (shaded)"=3711, "Left Pump (flat)"=3813, "Left Pump (shaded)"=3713, "Left Rect Valve (flat)"=3700, "Left Rect Valve (outline)"=3800, "Left Rect Valve (shaded)"=21760, "Left Tee (flat)"=3809, "Left Tee (shaded)"=3709, "Left Up Elbow (flat)"=3808, "Left Up Elbow (shaded)"=3708, "Less Or Equal To 0?"=1115, "Less Or Equal?"=1104, "Less Than 0?"=1118, "Less?"=1111, "Lexical Class"=1126, "Line (chiseled, system)"=3632, "Line (chiseled, thick)"=3630, "Line (chiseled, thin)"=3627, "Line (thick)"=3629, "Line (thin)"=3626, "Line Feed Constant"=23501, "Line with Arrow (thick)"=3631, "Line with Arrow (thin)"=3628, "List Directory"=1418, "List Folder"=8083, "Listbox (classic)"=21806, "Listbox (modern)"=21792, "Listbox (system)"=21805, "Listbox Symbol Ring Constant"=2038, "Load Certificates Into Memory"=1734, "Load Private Key Into Memory"=1733, "Local Variable"=2061, "Lock Range"=1411, "Logarithm Base 10"=1210, "Logarithm Base 2"=1225, "Logarithm Base X"=1224, "Logical Shift"=1081, "Look In Map"=2458, "Lookup Channel Probe"=9155, "Lossy Enqueue Element"=9130, "Lowered Box (thick)"=3635, "Lowered Rounded Box"=3638, "Machine Epsilon"=23528, "Make TLS Configuration Immutable"=1737, "MakeAddr"=1967, "Mantissa & Exponent"=1150, "Map"=3488, "Map Constant"=2461, "Match First String"=1532, "Match Pattern"=1535, "Match True/False String"=1533, "MathScript Call By Reference"=3906, "MathScript Node"=2357, "MATLAB script"=9020, "MATLAB Session Refnum"=3490, "Matrix Size"=8507, "Max & Min"=1108, "Menu Refnum"=3413, "Menu Ring (classic)"=3018, "Menu Ring (modern)"=21600, "Menu-Popup Ring"=3017, "Merge Errors"=2147, "Merge Signals"=2350, "Meter (classic)"=3030, "Meter (modern)"=21008, "Mixed Checkbox (system)"=21333, "Mixed Signal Graph"=21721, "Molar Gas Constant (J/(mol K))"=23522, "Motion Resource (block diagram constant)"=3449, "Motion Resource (classic)"=3448, "Motion Resource (modern)"=21787, "Motor (flat)"=3820, "Motor (shaded)"=3720, "Move"=8068, "Move (deprecated)"=1415, "Multi-Segment Pipe"=23780, "Multicolumn Listbox (classic)"=21799, "Multicolumn Listbox (modern)"=21791, "Multicolumn Listbox (system)"=21798, "Multiply"=1052, "Multiply (with error terminals)"=3917, "Multiply Array Elements"=1904, "Multirate Structure"=2199, "Natural Logarithm"=1209, "Natural Logarithm (Arg +1)"=1221, "Natural Logarithm Base"=23510, "Natural Logarithm Of 10"=23513, "Natural Logarithm Of 2"=23514, "Natural Logarithm Of Pi"=23508, "Negate"=1069, "Negative Infinity"=23509, "New Data Value Reference"=2408, "New Directory"=1402, "New File"=1404, "New TLS Configuration"=1730, "New VI"=8014, "New VI Object"=8015, "Not"=1064, "Not A Number/Path/Refnum?"=1128, "Not A Path Constant"=23524, "Not a Refnum Constant"=23526, "Not a Shared Variable"=23527, "Not And"=1071, "Not Equal To 0?"=1116, "Not Equal?"=1105, "Not Exclusive Or"=1073, "Not Or"=1072, "Notifier Refnum"=3423, "Number of Cache Levels"=24133, "Number To Boolean Array"=1814, "Number To Decimal String"=1180, "Number To Engineering String"=1183, "Number To Exponential String"=1505, "Number To Fractional String"=1506, "Number To Hexadecimal String"=1181, "Number To Octal String"=1182, "Numeric Constant"=2005, "Numeric Control (classic)"=3000, "Numeric Control (modern)"=21003, "Numeric Control (system)"=21919, "Numeric Indicator (classic)"=3001, "Numeric Indicator (modern)"=21004, "Obtain Notifier"=9101, "Obtain Queue"=9108, "Occurrence Refnum"=3406, "Octal Digit?"=1129, "Octal String To Number"=1186, "OK Button (modern)"=21738, "OK Button (system)"=3130, "Old VISA Open"=1921, "OLE Variant"=3150, "One Button Dialog"=1340, "Open and Verify Variable Connection"=23790, "Open Application Reference"=8012, "Open Device"=1430, "Open Dynamic Bitfile Reference"=5691, "Open File"=1403, "Open MATLAB Session"=24208, "Open Python Session"=24206, "Open Tank (flat classic)"=21752, "Open Tank (shaded classic)"=3074, "Open Variable Connection"=23779, "Open Variable Connection in Background"=23791, "Open VI Object Reference"=8013, "Open VI Reference"=8010, "Open/Create/Replace Datalog"=8054, "Open/Create/Replace File"=8050, "Or"=1062, "Or Array Elements"=1910, "Oval with Shadow"=32509, "Package Matrix"=23001, "PassControl"=1968, "Path Constant"=2009, "Path to Array of Strings"=1423, "Path To String"=1077, "Path Type"=1421, "Pi"=23504, "Pi Divided By 2"=23506, "Pi Multiplied By 2"=23505, "Pick Line"=1510, "Pict Ring (classic)"=3015, "Pict Ring (modern)"=21602, "Pict Ring (system)"=21925, "PixMap"=3505, "PixMap (warning: dangerous)"=3507, "Planck's Constant (J/Hz)"=23516, "Platform Flat Square Button"=3134, "Plug-In Control"=21820, "Polar To Complex"=1047, "Polar To Re/Im"=23061, "Positive Infinity"=23515, "Power Of 10"=1212, "Power Of 2"=1223, "Power Of X"=1213, "PPoll"=1969, "PPollConfig"=1970, "PPollUnconfig"=1971, "Preallocated Read from Binary File"=24135, "Preserve Run-Time Class"=8018, "Pressure Tank (flat)"=3075, "Pressure Tank (shaded)"=21753, "Preview Queue Element"=9112, "Printable?"=1124, "Property Node"=1920, "Pulldown Menu Ring"=3061, "Push Button"=21001, "Python Node"=24205, "Python Session Refnum"=3486, "Queue Refnum"=3424, "Quit LabVIEW"=1352, "Quotient & Remainder"=1056, "Race Structure"=2371, "Radio Button (system)"=3133, "Radio Buttons (classic)"=22003, "Radio Buttons (modern)"=22001, "Radio Buttons (system)"=22002, "Raised Box (classic)"=3600, "Raised Box (modern)"=3637, "Raised Circle"=3603, "Raised Down Triangle"=3615, "Raised Frame"=3606, "Raised Left Triangle"=3612, "Raised Right Triangle"=3613, "Raised Rounded Box"=3609, "Raised Up Triangle"=3614, "Random Number (0-1)"=1070, "RcvRespMsg"=1972, "Re-accept TLS"=1739, "Re/Im To Complex"=1046, "Re/Im To Polar"=23060, "Read Datalog"=8069, "Read Device"=1432, "Read File"=1407, "Read from Binary File"=8051, "Read from Text File"=8070, "Read Map Max & Min Keys"=2459, "Read Multiple Elements from Stream"=23803, "Read Set Max & Min"=2455, "Read Single Element from Stream"=23797, "Read Variable"=23781, "Read Variable with Timeout"=23786, "ReadStatus"=1973, "Receive"=1974, "ReceiveSetup"=1975, "Recessed Box"=3601, "Recessed Circle"=3604, "Recessed Down Triangle"=3619, "Recessed Frame (modern)"=3607, "Recessed Frame (system)"=3624, "Recessed Left Triangle"=3616, "Recessed Menu Ring"=3019, "Recessed Right Triangle"=3617, "Recessed Rounded Box"=3610, "Recessed Up Triangle"=3618, "Reciprocal"=1059, "Reciprocal Of e"=23511, "Reciprocal Of Pi"=23507, "RecomposeUnlockDataValRef (warning: dangerous)"=2407, "RecomposeVariant (warning: dangerous)"=2405, "Rectangular Stop Button"=3128, "Refnum to Path"=1424, "Refnum to Session"=2306, "Region"=2196, "Register Event Callback"=2078, "Register For Events"=2065, "Register Session"=2319, "Release Notifier"=9102, "Release Queue"=9109, "Remove Fixed-Point Overflow Status"=5563, "Remove From Map"=2457, "Remove From Set"=2453, "Replace Array Subset"=3910, "Replace Substring"=3913, "Request Deallocation"=1610, "ResetSys"=1976, "Reshape Array"=2055, "Resize Matrix"=8508, "Resource Index"=1088, "Reverse 1D Array"=1900, "Reverse String"=1537, "Right Arrow"=3825, "Right Bow Valve (flat)"=3705, "Right Bow Valve (outline)"=3805, "Right Bow Valve (shaded)"=21765, "Right Down Elbow (flat)"=3817, "Right Down Elbow (shaded)"=3717, "Right Pump (flat)"=3819, "Right Pump (shaded)"=3719, "Right Rect Valve (flat)"=3704, "Right Rect Valve (outline)"=3804, "Right Rect Valve (shaded)"=21764, "Right Tee (flat)"=3815, "Right Tee (shaded)"=3715, "Right Up Elbow (flat)"=3814, "Right Up Elbow (shaded)"=3714, "Rocker"=21002, "Rotary Feeder"=3830, "Rotate"=1082, "Rotate 1D Array"=1906, "Rotate Left With Carry"=1606, "Rotate Right With Carry"=1607, "Rotate String"=1536, "Round Button"=3100, "Round LED (classic)"=3120, "Round LED (modern)"=21012, "Round Light"=3104, "Round Push Button"=3118, "Round Push Button (profile)"=3112, "Round Radio Button"=3106, "Round Stop Button"=3127, "Round To Nearest"=1055, "Round Toward +Infinity"=1076, "Round Toward -Infinity"=1075, "Rounded Rectangle with Shadow"=32508, "RT FIFO Create"=24000, "RT FIFO Delete"=24003, "RT FIFO Read"=24001, "RT FIFO Write"=24002, "Rydberg Constant (1/m)"=23521, "Scale By Power Of 2"=1074, "Scan From File"=2082, "Scan From String"=2080, "Scan String For Tokens"=8101, "Scan Value"=1534, "Scanned Variable Read"=23784, "Scanned Variable Write"=23787, "Search 1D Array"=1901, "Search and Replace String"=3914, "Search Variable Container"=23802, "Search/Split String"=1538, "Secant"=1203, "Seconds To Date/Time"=1309, "Seek"=1409, "Select"=1516, "Send"=1977, "Send Notification"=9104, "SendCmds"=1978, "SendDataBytes"=1979, "SendIFC"=1980, "SendList"=1981, "SendLLO"=1982, "SendSetup"=1983, "Session to Refnum"=2307, "Set"=3487, "Set Constant"=2460, "Set Control Values by Index"=24203, "Set Datalog Position"=8072, "Set File Position"=8073, "Set File Size"=8074, "Set Matrix Diagonal"=8504, "Set Matrix Elements"=8505, "Set Menu Item Info"=9006, "Set Number of Records"=8075, "Set Occurrence"=1702, "Set Permissions"=8076, "Set Submatrix"=8506, "Set Type and Creator"=8077, "Set Variant Attribute"=8204, "Set Waveform Attribute"=8207, "SetRWLS"=1984, "SetTimeOut"=1985, "Shared Variable"=23778, "Shared Variable Constant"=3473, "Shared Variable Control (classic)"=3472, "Shared Variable Control (modern)"=21814, "Shared Variable to String"=1831, "Sign"=1049, "Simple Horizontal Slide"=3003, "Simple Numeric"=2900, "Simple String"=2115, "Simple Vertical Slide"=3002, "Sinc"=1227, "Sine"=1200, "Sine & Cosine"=1220, "Size Handle"=1603, "Slide Switch"=21011, "Smoothed Oval"=32500, "Smoothed Rounded Rectangle"=32505, "Sort 1D Array"=1120, "Sort Array of String"=23065, "Speed Of Light In Vacuum (m/sec)"=23518, "Spin Control (system)"=21900, "Split 1D Array"=1908, "Split Button"=21020, "Split Number"=1170, "Split Signals"=2351, "Spreadsheet String To Array"=1539, "Square"=23059, "Square Button"=3101, "Square LED (classic)"=3121, "Square LED (modern)"=21013, "Square Light"=3105, "Square Push Button"=3119, "Square Push Button (profile)"=3113, "Square Radio Button"=3107, "Square Root"=1060, "Stacked Sequence Structure"=2000, "Start TLS"=1731, "State"=2198, "State Diagram"=2051, "Static VI Reference"=2084, "Stop"=1350, "Stop Button"=21230, "String Constant"=2007, "String Control (classic)"=3200, "String Control (modern)"=21701, "String Control (system)"=21920, "String Indicator (classic)"=3201, "String Indicator (modern)"=21702, "String Length"=1502, "String Subset"=1503, "String To Byte Array"=1608, "String To IP"=1711, "String To Path"=1078, "String to Shared Variable"=1830, "Strip Path"=1420, "SubPanel"=21810, "SubPanel (Classic)"=21811, "SubPanel (NXG Style)"=21824, "SubPanel (System)"=21823, "Subtract"=1051, "Subtract (with error terminals)"=3916, "Swap Bytes"=1162, "Swap Values"=2401, "Swap Vector Element"=1912, "Swap Words"=1163, "Tab Constant"=23502, "Tab Control (classic)"=3330, "Tab Control (modern)"=3332, "Tab Control (NXG Style)"=32700, "Tab Control (system)"=3331, "Table (classic)"=21796, "Table (modern)"=21790, "Table (system)"=21797, "Tag Attribute Ring"=2063, "Tangent"=1202, "Tank (classic)"=3020, "Tank (modern)"=21006, "Target Structure"=2370, "TCP Close Connection"=1713, "TCP Create Listener"=1717, "TCP Flattened Read"=1718, "TCP Flattened Write"=1719, "TCP Flex Read"=1720, "TCP Flex Write"=1721, "TCP Network Connection Refnum"=3407, "TCP Open Connection"=1715, "TCP Read"=1716, "TCP Wait On Listener"=1712, "TCP Write"=1714, "TDMS Advanced Asynchronous Read (Data Ref)"=2151, "TDMS Advanced Asynchronous Write (Data Ref)"=2150, "TDMS Close"=24113, "TDMS Configure Asynchronous Reads (Data Ref)"=2153, "TDMS Configure Asynchronous Writes (Data Ref)"=2152, "TDMS Defragment"=24119, "TDMS Delete Data"=2159, "TDMS File"=3477, "TDMS Flush"=24117, "TDMS Get Asynchronous Read Status (Data Ref)"=2155, "TDMS Get Asynchronous Write Status (Data Ref)"=2154, "TDMS Get Properties"=24115, "TDMS In Memory Close"=2157, "TDMS In Memory Open"=2156, "TDMS In Memory Read Bytes"=2158, "TDMS List Contents"=24116, "TDMS Open"=24112, "TDMS Read"=24111, "TDMS Refnum To File ID"=24120, "TDMS Set Properties"=24114, "TDMS Write"=24110, "TDMS Write IP"=24118, "Temporary Directory"=1435, "TestSRQ"=1986, "TestSys"=1987, "Text & Pict Ring (classic)"=3016, "Text & Pict Ring (modern)"=21603, "Text Button"=21015, "Text Ring (block diagram constant)"=2008, "Text Ring (classic)"=3014, "Text Ring (modern)"=21601, "Text Ring (system)"=3060, "Text to UTF-8"=23066, "Thermometer (classic)"=3021, "Thermometer (modern)"=21007, "Threshold 1D Array"=1909, "Tick Count (ms)"=1300, "Time Stamp (block diagram constant)"=2068, "Time Stamp Control (classic)"=5555, "Time Stamp Control (modern)"=21913, "Time Stamp Control (system)"=21967, "Time Stamp Indicator (classic)"=5556, "Time Stamp Indicator (modern)"=21914, "Timed Loop"=5570, "Timed Sequence"=5573, "TLS configuration"=3489, "TLS Connection?"=1740, "To Byte Integer"=1140, "To Double Precision Complex"=1152, "To Double Precision Float"=1147, "To Extended Precision Complex"=1154, "To Extended Precision Float"=1149, "To Fixed-Point"=5561, "To Long Integer"=1142, "To Lower Case"=1189, "To More Generic Class"=8017, "To More Specific Class"=8016, "To OLE Variant"=8002, "To Probe String"=2413, "To Quad Integer"=1155, "To Single Precision Complex"=1151, "To Single Precision Float"=1146, "To Time Stamp"=5560, "To Unsigned Byte Integer"=1143, "To Unsigned Long Integer"=1145, "To Unsigned Quad Integer"=1156, "To Unsigned Word Integer"=1144, "To Upper Case"=1188, "To Variant"=8201, "To Word Integer"=1141, "Traditional DAQ Channel (block diagram constant)"=2085, "Traditional DAQ Channel (classic)"=3320, "Traditional DAQ Channel (modern)"=21733, "Transpose 1D Array"=23068, "Transpose 2D Array"=1902, "Transpose Matrix"=8509, "Tree (classic)"=21819, "Tree (modern)"=21793, "Tree (system)"=21794, "Trigger"=1988, "TriggerList"=1989, "Two Button Dialog"=1341, "Type and Creator"=1434, "Type Cast"=1166, "Type Error"=2415, "Type Must Be Array"=2417, "Type Must Be Cluster"=2418, "Type Of"=2414, "Type Specialization Structure"=2373, "UDP Close"=1726, "UDP Multicast Open"=1727, "UDP Network Connection Refnum"=3418, "UDP Open"=1723, "UDP Read"=1724, "UDP Write"=1725, "Unbitpack from Array"=3136, "Unbundle"=2048, "Unbundle By Name"=2058, "Unflatten From JSON"=24202, "Unflatten From String"=1165, "Unflatten From XML"=8401, "Unleak Variant Value Reference"=2411, "Unpackage Matrix"=23000, "Unregister For Events"=2076, "Unregister Session"=2320, "Up Arrow"=3823, "Up Bow Valve (flat)"=3703, "Up Bow Valve (outline)"=3803, "Up Bow Valve (shaded)"=21763, "Up Rect Valve (flat)"=3702, "Up Rect Valve (outline)"=21762, "Up Rect Valve (shaded)"=3802, "Up Tee (flat)"=3812, "Up Tee (shaded)"=3712, "User Defined Refnum"=3428, "User Defined Refnum Tag (block diagram constant)"=3426, "User Defined Refnum Tag (classic)"=3429, "User Defined Refnum Tag (modern)"=21745, "User Defined Refnum Tag Flatten (classic)"=3454, "User Defined Refnum Tag Flatten (modern)"=21747, "User Defined Tag (block diagram constant)"=2114, "User Defined Tag (classic)"=3329, "User Defined Tag (modern)"=21749, "User Item"=3506, "UTF-8 String To Byte Array"=1650, "UTF-8 to Text"=23067, "Variable Class Specifier Constant"=2106, "Variable Name Constant"=3478, "Variant"=3310, "Variant To Data"=8003, "Variant To Flattened String"=8203, "Vert Line"=3822, "Vert Pipe (flat)"=3816, "Vert Pipe (shaded)"=3716, "Vert Rocker"=21740, "Vertical Fill Slide (classic)"=3009, "Vertical Fill Slide (modern)"=21014, "Vertical Gradient Oval"=32501, "Vertical Gradient Rectangle"=32503, "Vertical Gradient Rounded Rectangle"=32506, "Vertical Graduated Bar"=21107, "Vertical Pointer Slide (classic)"=3007, "Vertical Pointer Slide (modern)"=21017, "Vertical Pointer Slide (system)"=21901, "Vertical Progress Bar (modern)"=21104, "Vertical Progress Bar (system)"=21909, "Vertical Scrollbar"=21111, "Vertical Slide (system)"=21903, "Vertical Slide Switch (classic)"=3115, "Vertical Slide Switch (modern)"=21741, "Vertical Smooth Box"=3634, "Vertical Splitter Bar"=21860, "Vertical Splitter Bar (Classic)"=21862, "Vertical Splitter Bar (NXG Style)"=21866, "Vertical Splitter Bar (System)"=21864, "Vertical Switch"=3109, "Vertical Toggle Switch (classic)"=3111, "Vertical Toggle Switch (modern)"=21005, "VI Library"=1425, "VI Refnum"=3422, "VI Server Reference"=2091, "VISA Assert Interrupt Signal"=2309, "VISA Assert Trigger"=1929, "VISA Assert Utility Signal"=2310, "VISA Clear"=1927, "VISA Close"=1922, "VISA Disable Event"=1940, "VISA Discard Events"=1941, "VISA Enable Event"=1942, "VISA Find Resource"=1923, "VISA Flush I/O Buffer"=2302, "VISA GPIB Command"=2315, "VISA GPIB Control ATN"=2316, "VISA GPIB Control REN"=2304, "VISA GPIB Pass Control"=2317, "VISA GPIB Send IFC"=2318, "VISA In 16"=1930, "VISA In 32"=1944, "VISA In 64"=2140, "VISA In 8"=1936, "VISA Lock"=1993, "VISA Map Address"=1932, "VISA Map Trigger"=2311, "VISA Memory Allocation"=1997, "VISA Memory Allocation Ex"=2146, "VISA Memory Free"=1998, "VISA Move"=2303, "VISA Move In 16"=1948, "VISA Move In 32"=1991, "VISA Move In 64"=2144, "VISA Move In 8"=1946, "VISA Move Out 16"=1949, "VISA Move Out 32"=1992, "VISA Move Out 64"=2145, "VISA Move Out 8"=1947, "VISA Open"=2308, "VISA Out 16"=1931, "VISA Out 32"=1945, "VISA Out 64"=2141, "VISA Out 8"=1937, "VISA Peek 16"=1934, "VISA Peek 32"=1995, "VISA Peek 64"=2142, "VISA Peek 8"=1938, "VISA Poke 16"=1935, "VISA Poke 32"=1996, "VISA Poke 64"=2143, "VISA Poke 8"=1939, "VISA Read"=1925, "VISA Read STB"=1928, "VISA Read To File"=2313, "VISA Refnum to Session"=2300, "VISA Resource Name"=3421, "VISA resource name (classic)"=3409, "VISA resource name (modern)"=21737, "VISA Set I/O Buffer Size"=2301, "VISA Status Description"=1924, "VISA Unlock"=1994, "VISA Unmap Address"=1933, "VISA Unmap Trigger"=2312, "VISA USB Control In"=2086, "VISA USB Control Out"=2087, "VISA VXI Cmd or Query"=2305, "VISA Wait on Event"=1943, "VISA Write"=1926, "VISA Write From File"=2314, "Volume Info"=1414, "Wait (ms)"=1302, "Wait For Activity"=1722, "Wait For Front Panel Activity"=1328, "Wait for GPIB RQS"=1952, "Wait on Notification"=9105, "Wait on Notification from Multiple"=9106, "Wait on Notification from Multiple with Notifier History"=9132, "Wait on Notification with Notifier History"=9131, "Wait on Occurrence"=1701, "Wait Until Next ms Multiple"=1327, "WaitSRQ"=1990, "Waveform Chart"=21010, "Waveform Chart (classic)"=3501, "Waveform Chart (modern)"=21717, "Waveform Graph (classic)"=3504, "Waveform Graph (modern)"=21703, "While Loop #1"=2003, "While Loop #2"=2352, "White Space?"=1125, "Write Datalog"=8079, "Write Device"=1431, "Write File"=1408, "Write Multiple Elements to Stream"=23804, "Write Single Element to Stream"=23798, "Write to Binary File"=8078, "Write to Text File"=8080, "Write Variable"=23782, "Write Variable with Timeout"=23789, "XY Graph (classic)"=3500, "XY Graph (modern)"=21716, "Y-th Root of X"=23062]
                        n151 = invoke class="Wire" method="Insert Node"(reference=w358, "Style"=w352, "PaletteString"=w354, "InsertPoint"=w351) -> (reference out=w355:refnum<vi>, error out=w353:errorcluster, "Insert Node"=w356:refnum<vi>)  [unwired: 3 in, 4 out]
                        n152 = call <vilib>:"Insert_Fix Node Terminals.vi"("Inserted Node"=w356, "error in (no error)"=w353, "Original Wire"=w355, "Node Name"=w354) -> ("error out"=w357:errorcluster)  [unwired: 7 in]
                      }
                      frame "" {
                        n153 = invoke class="Wire" method="Insert Node"(reference=w363, "Path"=w362, "InsertPoint"=w359) -> (error out=w361:errorcluster, "Insert Node"=w360:refnum<vi>)  [unwired: 4 in, 5 out]
                      }
                    }
                  }
                  frame False {
                    n154 = case shown="Default" w369 {
                      selector: w369 -> [w371 _]
                      tunnel: w366 -> [w376 w381]
                      tunnel: w368 -> [_ w380]
                      tunnel: [w374 w379] -> w365
                      tunnel: [w373 w378] -> w367
                      tunnel: w364 -> [w370 w377]
                      frame Default {
                        n155 = invoke class="Wire" method="Insert Node"(reference=w376, "PaletteString"=w371, "InsertPoint"=w370) -> (reference out=w372:refnum<vi>, error out=w375:errorcluster, "Insert Node"=w373:refnum<vi>)  [unwired: 4 in, 4 out]
                        n156 = call <vilib>:"Insert_Fix Node Terminals.vi"("Inserted Node"=w373, "error in (no error)"=w375, "Original Wire"=w372, "Node Name"=w371) -> ("error out"=w374:errorcluster)  [unwired: 7 in]
                      }
                      frame "" {
                        n157 = invoke class="Wire" method="Insert Node"(reference=w381, "Path"=w380, "InsertPoint"=w377) -> (error out=w379:errorcluster, "Insert Node"=w378:refnum<vi>)  [unwired: 4 in, 5 out]
                      }
                    }
                  }
                }
                n158 = Not(x=w339) -> (.not. x?=w338:bool)
              }
              n159 = Or Array Elements(Boolean array=w331) -> (logical OR=w330:bool)
              n160 = for {
                tunnel: w329 -> [w383] mode=indexing
                shift-right: [w385] -> _
                shift-left: T2[] [] -> [w384]
                n161 = Not A Number/Path/Refnum?(number/path/refnum=w383) -> (NaN/Path/Refnum?=w382:bool)
                n162 = case shown="False" w382 {
                  tunnel: w383 -> [w391 _]
                  tunnel: [w390 w426] -> w385
                  tunnel: w384 -> [w388 w426]
                  frame False {
                    # "See if current item's position is within 5 pixels of any other item's position."
                    n163 = property class="GObj"(reference=w391) -> (reference out=w389:refnum<vi>, "Position"=w387:T2)  [unwired: 1 in, 1 out]
                    n164 = for {
                      tunnel: w388 -> [w400] mode=indexing
                      tunnel: w387 -> [w396]
                      tunnel: [w392] -> w386
                      stop <- w392 stop-if-true
                      w399 = 5 ("y")
                      n165 = Add(x=w400, y=w399) -> (x+y=w398:T2)
                      n166 = Subtract(x=w400, y=w399) -> (x-y=w397:T2)
                      n167 = In Range and Coerce(upper limit=w398, x=w396, lower limit=w397) -> (In Range?=w395:cluster{"Left":bool, "Top":bool})  [unwired: 1 out]
                      n168 = Unbundle(w395) -> ("Left"=w394:bool, "Top"=w393:bool)
                      n169 = And(x=w394, y=w393) -> (x .and. y?=w392:bool)
                    }
                    n170 = case shown="True" w386 {
                      tunnel: w388 -> [w404 w425]
                      tunnel: [w403 w424] -> w390
                      tunnel: w387 -> [w402 w423]
                      tunnel: w389 -> [w405 _]
                      frame True {
                        # "This object position exists (within 5 pixels of another object). Add 5 pixels to h/v until a position is found that does not overlap (with 5 pixels), and use that."
                        n171 = while {
                          tunnel: w404 -> [w408]
                          tunnel: w402 -> [w409]
                          tunnel: [w407] -> w401
                          i -> [w413]
                          stop <- w406 continue-if-true
                          # "See if current item's position is within 5 pixels of any other item's position."
                          n172 = Increment(x=w413) -> (x+1=w412:i32)
                          n173 = Multiply(x=5 ("y"), y=w412) -> (x*y=w410:i32)
                          n174 = Add(x=w409, y=w410) -> (x+y=w407:T2)
                          n175 = for {
                            tunnel: w408 -> [w422] mode=indexing
                            tunnel: w407 -> [w418]
                            tunnel: [w414] -> w406
                            stop <- w414 stop-if-true
                            w421 = 5 ("y")
                            n176 = Add(x=w422, y=w421) -> (x+y=w420:T2)
                            n177 = Subtract(x=w422, y=w421) -> (x-y=w419:T2)
                            n178 = In Range and Coerce(upper limit=w420, x=w418, lower limit=w419) -> (In Range?=w417:cluster{"Left":bool, "Top":bool})  [unwired: 1 out]
                            n179 = Unbundle(w417) -> ("Left"=w416:bool, "Top"=w415:bool)
                            n180 = And(x=w416, y=w415) -> (x .and. y?=w414:bool)
                          }
                        }
                        n181 = property class="GObj"(reference=w405, "Position"=w401) -> ()  [unwired: 1 in, 2 out]
                        n182 = Build Array (concatenate)(w404, w401) -> (w403:T2[])
                      }
                      frame False {
                        # "This object's position doesn't exist in the array. Store it to compare with later objects."
                        n183 = Build Array (concatenate)(w425, w423) -> (w424:T2[])
                      }
                    }
                  }
                  frame True {
                    # "Invalid refnum...don't bother doing anything"
                  }
                }
              }
              n184 = Index Array(array=w329) -> (element=→"element":refnum<vi>)  [unwired: 1 in]
            }
          }
        }
        frame True {
        }
      }
    }
    frame Error {
    }
  }
  "error out" <- w7
  "Variant out" <- w3
